vi "handle-error.vi"(8 "error in (no error)":errorcluster, 10 "state-in":T1) -> (0 "error out":errorcluster, 2 "state":T1)   [LabVIEW 2017, in "Library.lvlib"]
uses:
  Library.lvlib
  state.ctl
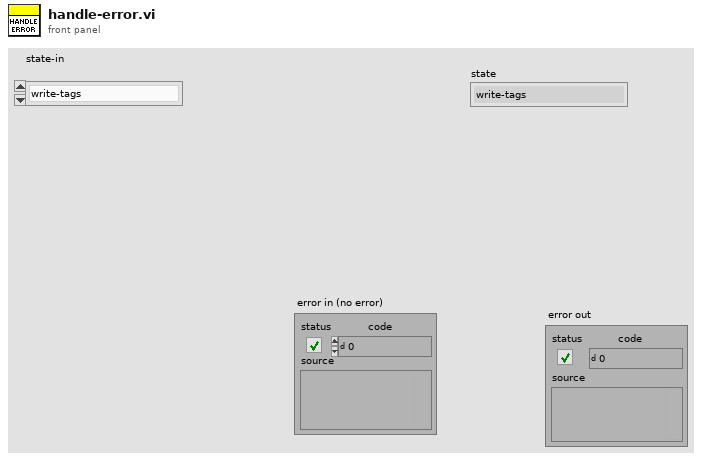
[diagram p1: front panel]
types:
  T1 = typedef "Library.lvlib/state.ctl" = enum16{"write-tags", "clear-fault", "generate-fault", "handle-error"}
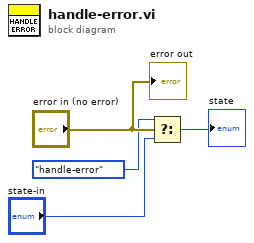
[diagram p0: block diagram]
diagram:
  n1 = Select(t=state."handle-error" ("Enum"), s="error in (no error)", f="state-in") -> (s? t:f=→"state":T1)
  "error out" <- "error in (no error)"
